vi "Check Parent Actor.vi"(10 "Actor":refnum<class "Actor.lvclass">) -> (2 "Error":errorcluster)   [LabVIEW 2020, in "jettl.lvlib"]
uses:
  jettl.lvlib
  Actor/Actor.lvclass
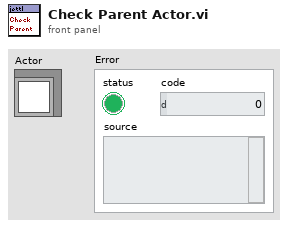
[diagram p1: front panel]
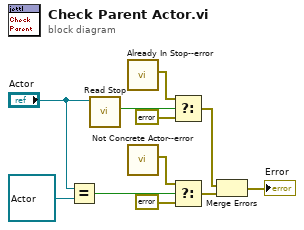
[diagram p0: block diagram]
diagram:
  n1 = Equal?(x="Actor", y=refnum<class "Actor.lvclass"> refnum ("jettl.lvlib:Actor.lvclass")) -> (x = y?=w5:bool)
  n2 = call-dynamic "Read Stop.vi"("Actor in"="Actor") -> ("Stop"=w9:bool)  [unwired: 10 in]
  n3 = call "Already In Stop--error.vi"() -> ("Error"=w11:errorcluster)  [unwired: 11 in]
  n4 = call "Not Concrete Actor--error.vi"() -> ("Error"=w6:errorcluster)  [unwired: 11 in]
  n5 = Select(t=w11, s=w9, f=errorcluster {"status"=FALSE, "code"=0, "source"=""}) -> (s? t:f=w3:errorcluster)
  n6 = Select(t=w6, s=w5, f=errorcluster {"status"=FALSE, "code"=0, "source"=""}) -> (s? t:f=w2:errorcluster)
  n7 = Merge Errors(w3, w2) -> (→"Error":errorcluster)
